vi "XLP80_CAN_Globals.vi"() -> ()   [LabVIEW 2021]
uses:
  XLP80_CAN/1886_PEAK_TDefEnumCANState.ctl
panel:
  out "Index Write Alarm":i32[](array[numeric])
  out "Index Read Alarm":i32[](array[numeric])
  out "Index Write Shutdown":i32[](array[numeric])
  out "Index Read Shutdown":i32[](array[numeric])
  out "Index Write Operational Mode":i32[](array[numeric])
  out "Index Read Operational Mode":i32[](array[numeric])
  out "Index WritePreconditions":i32[](array[numeric])
  out "Index WriteTestmodeA":i32[](array[numeric])
  out "Index Read TestmodeA":i32[](array[numeric])
  out "CounterCAN_WriteError":i32
  out "Index Write Power Management":i32[](array[numeric])
  out "Index Read Power Management":i32[](array[numeric])
  out "Index Write Basis Funktion":i32[](array[numeric])
  out "Index Read Basis Funktion":i32[](array[numeric])
  in  "IgnoreList":string[](array[string])
  out "Index Write HV&Software":i32[](array[numeric])
  out "Index Read HV&Software":i32[](array[numeric])
  in  "CAN State":T1
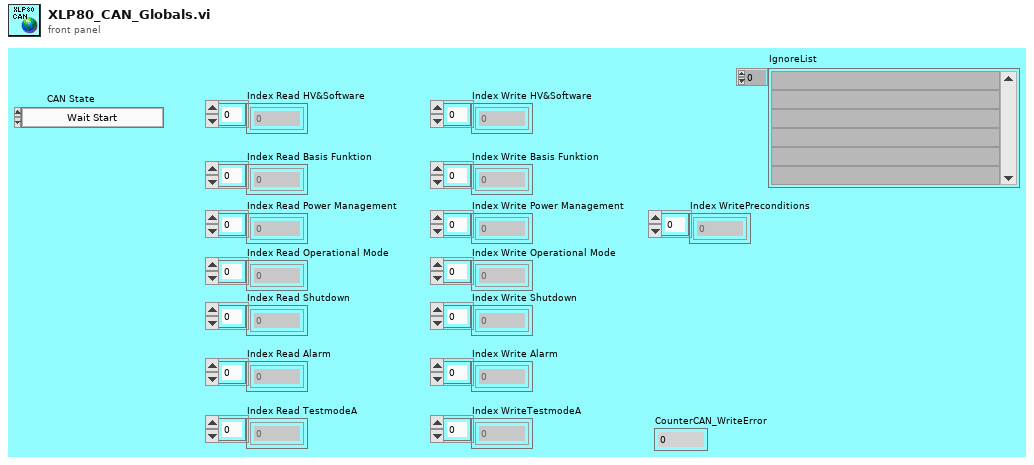
[diagram p1: front panel]
types:
  T1 = typedef "1886_PEAK_TDefEnumCANState.ctl" = enum16{"Wait Start", "Start CAN", "Run CAN", "Stop CAN"}
diagram:
